vi "Perfetto PPL Post-Build Action.vi"(5 "Files Generated by Build":path[](array[path]), 6 "Top Level/Always Included VIs":path[](array[path]), 7 "Destination Path":path, 8 "error in":errorcluster, 9 "Target Name":string, 10 "Build Specification Name":string, 11 "Project Path":path) -> (0 "error out":errorcluster)   [LabVIEW 2023]
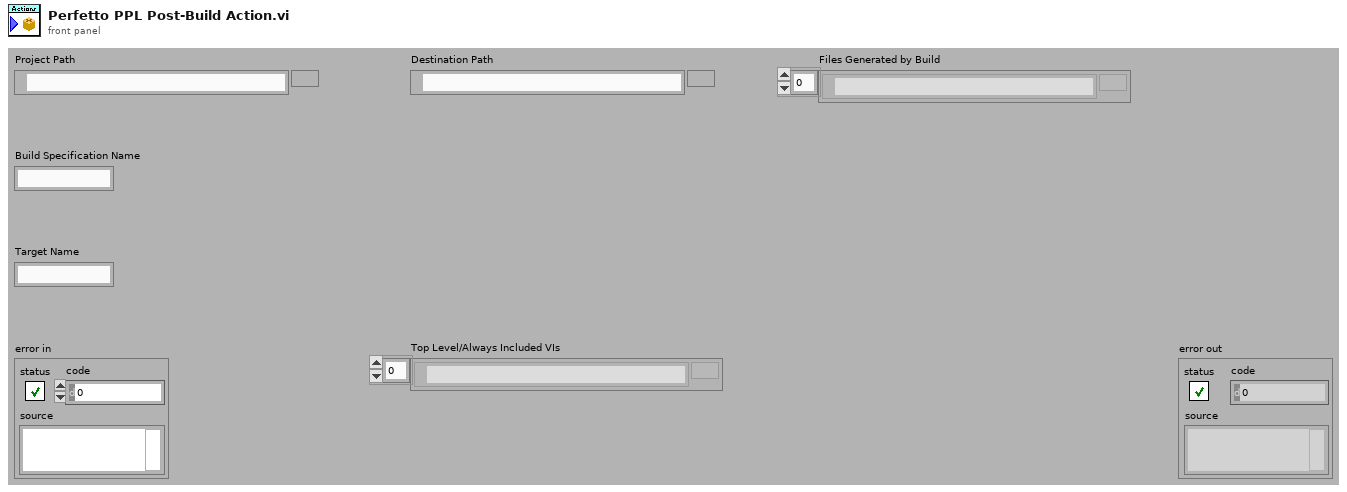
[diagram p1: front panel]
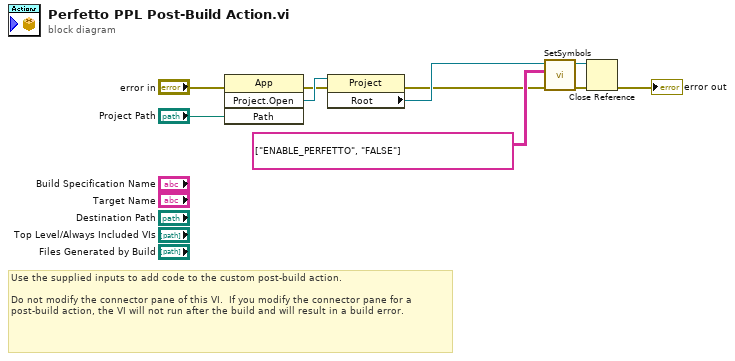
[diagram p0: block diagram]
diagram:
  # "Use the supplied inputs to add code to the custom post-build action.\n\nDo not modify the connector pane of this VI.  If you modify the connector pane for a post-build action, the VI will not run after the build and will result in a build error."
  n1 = invoke class="App" method="Project.Open"(error in="error in", "Path"="Project Path") -> (error out=w3:errorcluster, "Project:Open"=w9:refnum<vi>)  [unwired: 2 in, 2 out]
  n2 = property class="Project"(reference=w9, error in=w3) -> (error out=w2:errorcluster, "Root"=w8:refnum<vi>)  [unwired: 1 out]
  n3 = call <resource>:"SetSymbols.vi"("error in"=w2, "Symbol Value Pairs"=string[][] [["ENABLE_PERFETTO", "FALSE"]], "Project Item"=w8) -> ("error out"=w5:errorcluster, "Project Item"=w6:refnum<vi>)  [unwired: 7 in]
  n4 = Close Reference(reference=w6, error in (no error)=w5) -> (error out=→"error out":errorcluster)
